vi "Configure Form Object.vi"(8 "error in (no error)":errorcluster, 10 "Table Name":string, 11 "Form Model in":refnum<class "Form Model.lvclass">) -> (0 "error out":errorcluster, 2 "Form":refnum<class "Basic Form.lvclass">, 3 "Form Model out":refnum<class "Form Model.lvclass">)   [LabVIEW 2020]
uses:
  Database OOP/Table Libraries/Basic Form/Basic Form.lvclass
  Form Model.lvclass
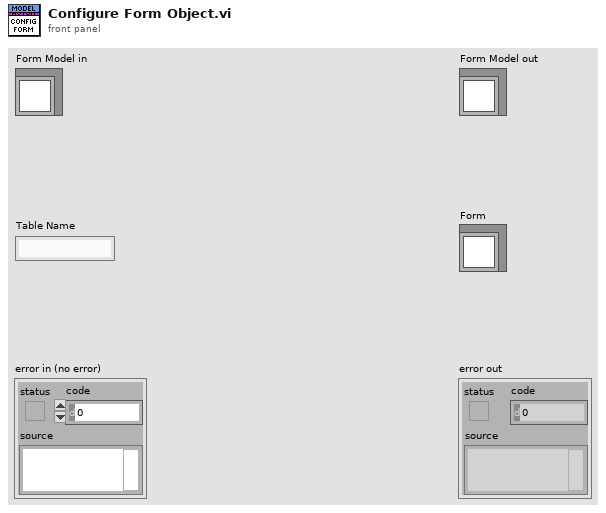
[diagram p1: front panel]
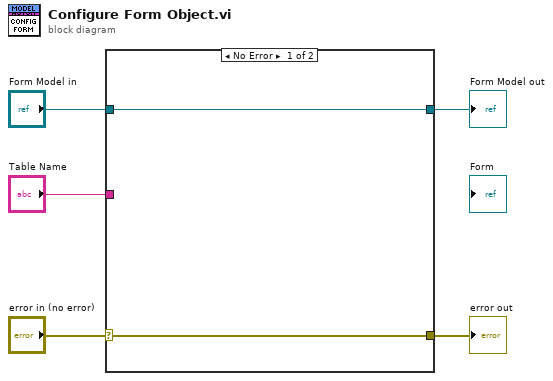
[diagram p0: block diagram]
diagram:
  n1 = case shown="No Error" "error in (no error)" {
    selector: "error in (no error)" -> [w7 w9]
    tunnel: "Form Model in" -> [w6 w8]
    tunnel: [w7 w9] -> w3
    tunnel: [w6 w8] -> w2
    tunnel: "Table Name" -> [_ _]
    frame No Error {
    }
    frame Error {
    }
  }
  "error out" <- w3
  "Form Model out" <- w2
